vi "Add A Directory.vi"(7 "Parrent":string, 10 "Name":string, 11 "Map":T1) -> (2 "Dir Name Out":string, 3 "Map Out":T1)   [LabVIEW 2020]
uses:
  MAP_Structure.ctl
  Cluster_Item Data.ctl
  <vilib>/Utility/miscctls.llb/LVMapReplaceAction.ctl
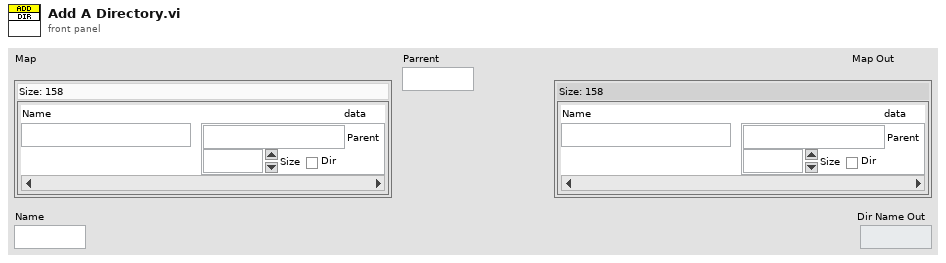
[diagram p1: front panel]
types:
  T1 = typedef "MAP_Structure.ctl" = map{string, T2}
  T2 = typedef "Cluster_Item Data.ctl" = cluster{"Parent":string, "Size":u32, "Dir":bool}
  T3 = typedef "LVMapReplaceAction.ctl" = enum32{"Modify Entry only if found", "Add or Modify Entry", "Delete Entry"}
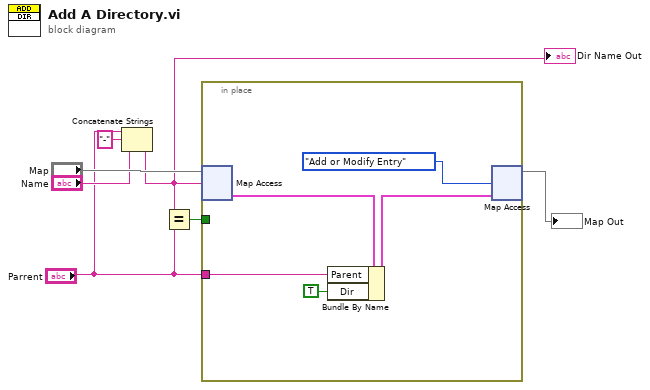
[diagram p0: block diagram]
diagram:
  n1 = Concatenate Strings("Parrent", "-" ("string"), "Name") -> (w4:string)
  "Dir Name Out" <- w4
  n2 = Equal?(x=w4, y="Parrent") -> (x = y?=w3:bool)
  n3 = in-place {
    in-place-border: "Parrent" -> [w9]
    in-place-border: w3 -> [_]
    n4 = in-place-map #1("Map", w4) -> (w11:T2)  [unwired: 1 in, 1 out]
    n5 = Bundle By Name(cluster=w11, "Parent"=w9, "Dir"=TRUE) -> (w10:T2)
    n6 = in-place-map #1(w10, LVMapReplaceAction."Add or Modify Entry" ("action")) -> (→"Map Out":T1)  [unwired: 2 out]
  }
